vi "PC Fish Control.vi"() -> ()   [LabVIEW 2014]
uses:
  <vilib>/Instr/_visa.llb/VISA Flush IO Buffer Mask.ctl
panel:
  in  "Tab Control":T1(tab)
  in  "Fish Communication Network\nVISA Port":refnum<visa-resource-name>="COM6"
  in  "GPS Network\nVISA Port":refnum<visa-resource-name>="COM8"
  in  "Fish Communication Network\nError In":errorcluster
  in  "GPS Network\nError In":errorcluster
  out "GPS Network \nHandshake Successful?":bool
  out "Comms Network \nHandshake Successful?":bool
  out "Handshake Complete":bool
  out "Handshake Aborted":bool
  in  "MHeading":i32(slide) scale=-45.0..45.0
  in  "MSpeed":i32(slide) scale=-50.0..50.0
  in  "Command Selection":string(combo)="0"
  out "Currently Transmitting\nComms Input":string
  in  "GPS Input":string="C, 400, 300 175"
  out "Currently Transmitting \nGPS Input":string
  out "Running?":bool
  in  "stop":bool caption="ESTOP"
  out "error out":errorcluster
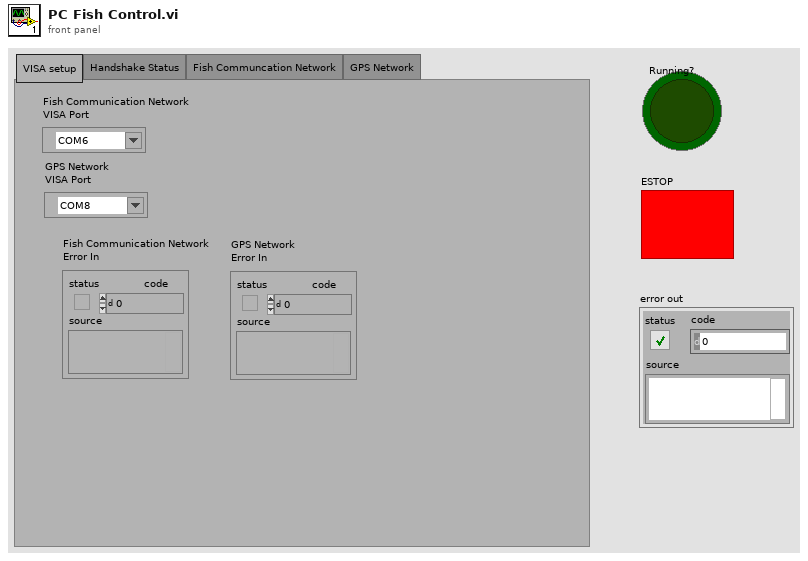
[diagram p1: front panel]
types:
  T1 = enum32{"VISA setup", "Handshake Status", "Fish Communcation Network", "GPS Network"}
  T2 = typedef "VISA Flush IO Buffer Mask.ctl" = u16
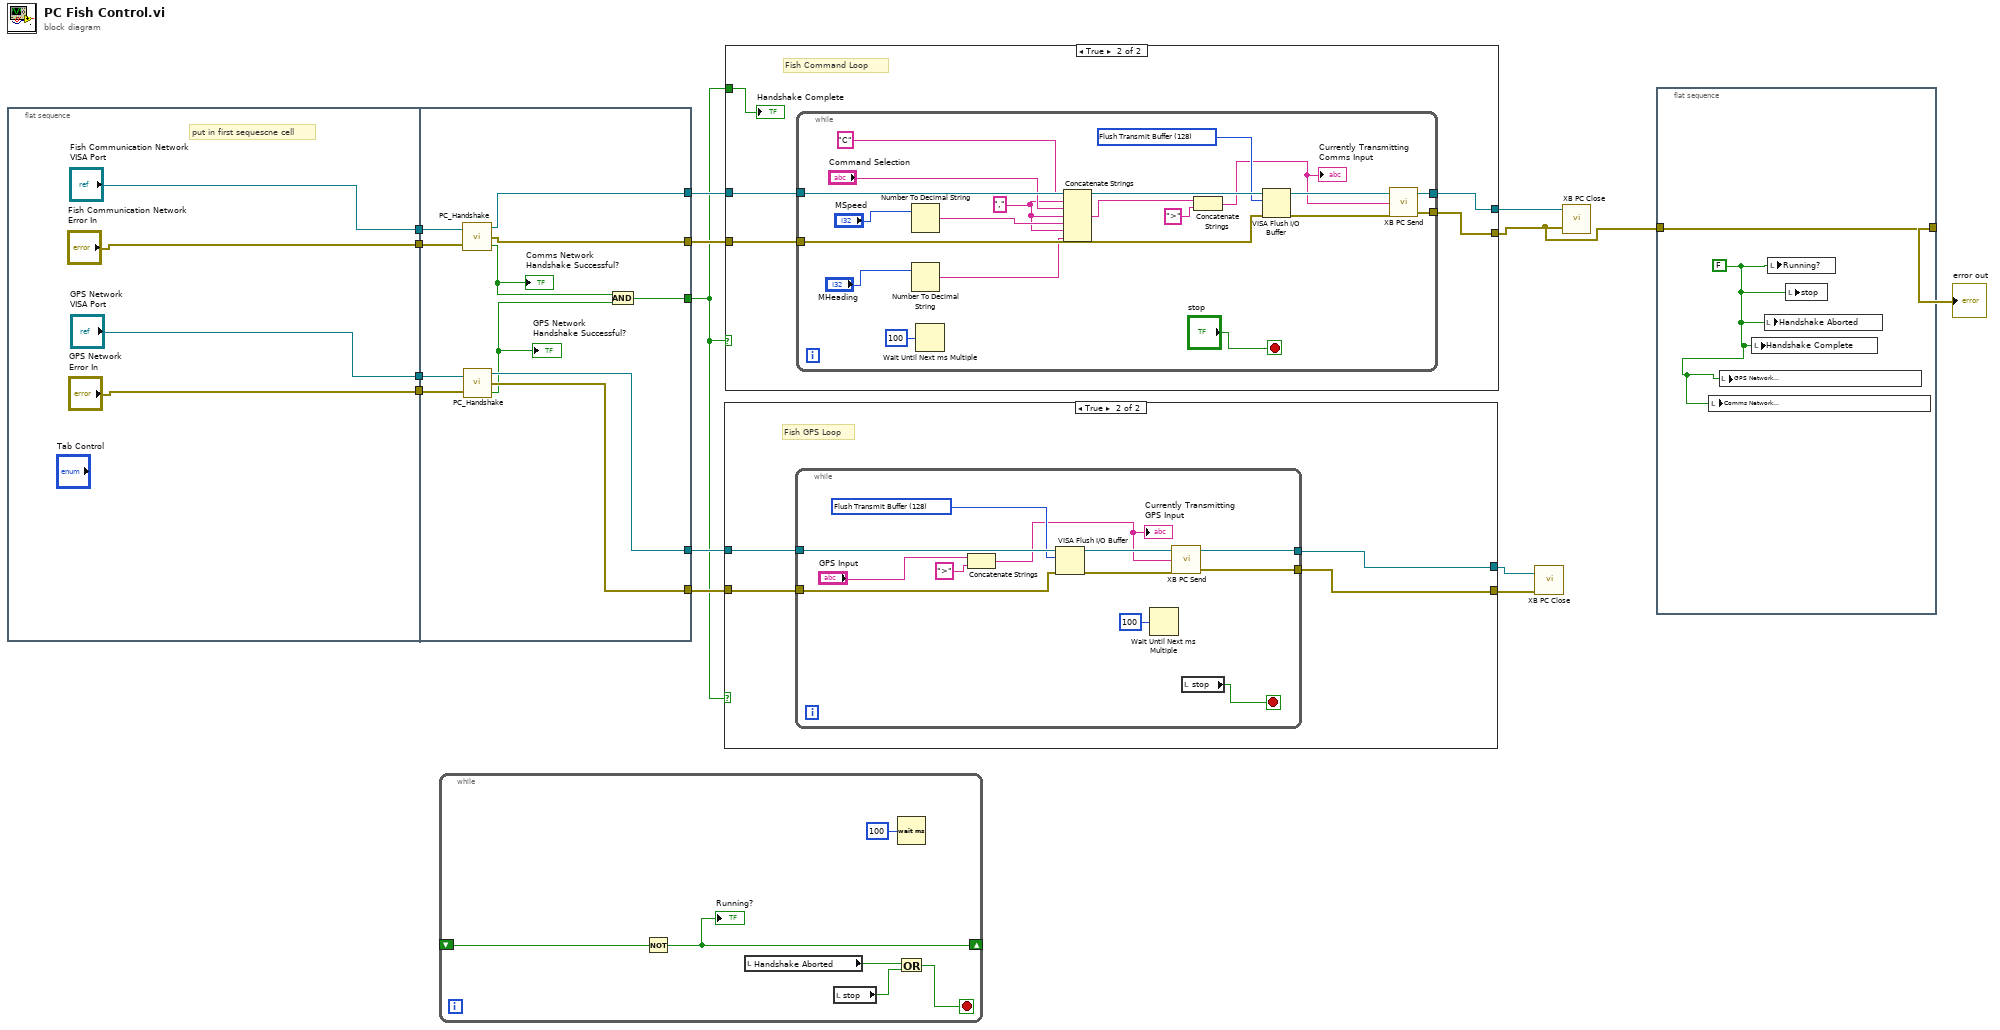
[diagram p0: block diagram]
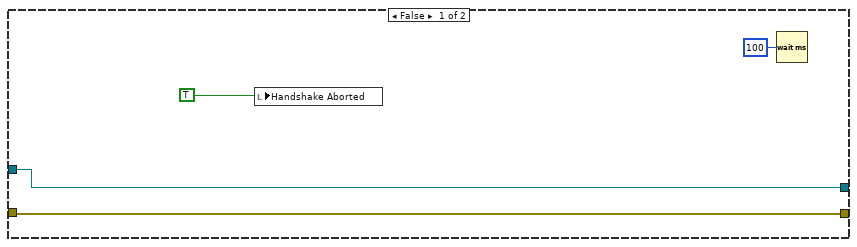
[diagram p2: hidden frame]
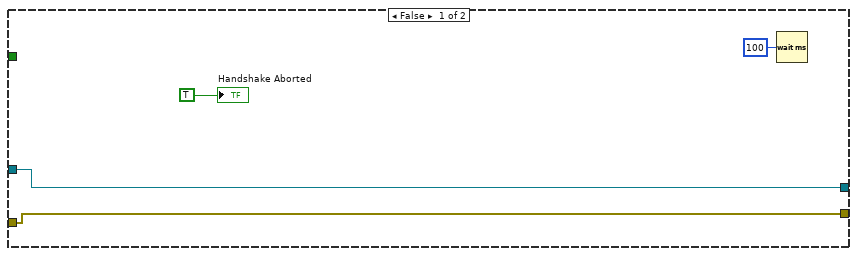
[diagram p3: hidden frame]
diagram:
  n1 = flat-sequence {
    tunnel: ["Fish Communication Network\nVISA Port"] -> w9
    tunnel: ["Fish Communication Network\nError In"] -> w8
    tunnel: ["GPS Network\nVISA Port"] -> w7
    tunnel: ["GPS Network\nError In"] -> w6
    tunnel: w9 -> [w29]
    tunnel: w8 -> [w28]
    tunnel: w7 -> [w27]
    tunnel: w6 -> [w26]
    tunnel: [w25] -> w5
    tunnel: [w24] -> w4
    tunnel: [w23] -> w3
    tunnel: [w22] -> w2
    tunnel: [w21] -> w1
    frame #0 {
      # "put in first sequescne cell"
    }
    frame #1 {
      n2 = call "PC_Handshake.vi"("VISA resource name"=w29, "error in"=w28) -> ("VISA resource name out"=w25:refnum<visa-resource-name>, "error out"=w24:errorcluster, "Handshake Successful?"=w19:bool)
      "Comms Network \nHandshake Successful?" <- w19
      n3 = call "PC_Handshake.vi"("VISA resource name"=w27, "error in"=w26) -> ("VISA resource name out"=w23:refnum<visa-resource-name>, "error out"=w22:errorcluster, "Handshake Successful?"=w20:bool)
      "GPS Network \nHandshake Successful?" <- w20
      n4 = And(x=w19, y=w20) -> (x .and. y?=w21:bool)
    }
  }
  n5 = while {
    shift-right: [w34] -> _
    shift-left: _ -> [w35]
    stop <- w32 stop-if-true
    n6 = Not(x=w35) -> (.not. x?=w34:bool)
    "Running?" <- w34
    n7 = local read "Handshake Aborted"() -> (w30:bool)
    n8 = local read "stop"() -> (w31:bool)
    n9 = Wait (ms)(milliseconds to wait=u32 100) -> ()  [unwired: 1 out]
    n10 = Or(x=w30, y=w31) -> (x .or. y?=w32:bool)
  }
  n11 = case shown="True" w1 {
    tunnel: w3 -> [w38 w43]
    tunnel: w2 -> [w37 w42]
    tunnel: [w38 w41] -> w12
    tunnel: [w37 w40] -> w11
    frame False {
      n12 = local write "Handshake Aborted"(TRUE) -> ()
      n13 = Wait (ms)(milliseconds to wait=u32 100) -> ()  [unwired: 1 out]
    }
    frame True {
      # "Fish GPS Loop"
      n14 = while {
        tunnel: w43 -> [w52]
        tunnel: w42 -> [w50]
        tunnel: [w53] -> w40
        tunnel: [w54] -> w41
        stop <- w45 stop-if-true
        w48 = T2 128 items=["Flush Receive Buffer"=16, "Write Transmit Buffer to Device"=32, "Flush Receive Buffer (No I/O)"=64, "Flush Transmit Buffer"=128] ("Mask")
        n15 = Concatenate Strings("GPS Input", ">" ("string")) -> (w46:string)
        "Currently Transmitting \nGPS Input" <- w46
        n16 = VISA Flush I/O Buffer(VISA resource name=w52, mask (16)=w48, error in (no error)=w50) -> (VISA resource name out=w51:refnum<visa-resource-name>, error out=w49:errorcluster)
        n17 = Wait Until Next ms Multiple(millisecond multiple=u32 100) -> ()  [unwired: 1 out]
        n18 = call "XB PC Send.vi"("error in (no error)"=w49, "String"=w46, "VISA resource name"=w51) -> ("error out"=w53:errorcluster, "VISA resource name out"=w54:refnum<visa-resource-name>)  [unwired: 1 out]
        n19 = local read "stop"() -> (w45:bool)
      }
    }
  }
  n20 = case shown="True" w1 {
    tunnel: w5 -> [w57 w64]
    tunnel: w1 -> [_ w61]
    tunnel: [w57 w63] -> w14
    tunnel: [w56 w62] -> w10
    tunnel: w4 -> [w56 w60]
    frame False {
      n21 = Wait (ms)(milliseconds to wait=u32 100) -> ()  [unwired: 1 out]
      "Handshake Aborted" <- TRUE
    }
    frame True {
      # "Fish Command Loop"
      n22 = while {
        tunnel: w64 -> [w79]
        tunnel: w60 -> [w77]
        tunnel: [w80] -> w62
        tunnel: [w81] -> w63
        stop <- "stop" stop-if-true
        w65 = "," ("string")
        w75 = T2 128 items=["Flush Receive Buffer"=16, "Write Transmit Buffer to Device"=32, "Flush Receive Buffer (No I/O)"=64, "Flush Transmit Buffer"=128] ("Mask")
        n23 = Number To Decimal String(number="MSpeed") -> (decimal integer string=w68:string)  [unwired: 1 in]
        n24 = Number To Decimal String(number="MHeading") -> (decimal integer string=w67:string)  [unwired: 1 in]
        n25 = Wait Until Next ms Multiple(millisecond multiple=u32 100) -> ()  [unwired: 1 out]
        n26 = Concatenate Strings("C" ("string"), w65, "Command Selection", w65, w68, w65, w67) -> (w69:string)
        n27 = Concatenate Strings(w69, ">" ("string")) -> (w74:string)
        "Currently Transmitting\nComms Input" <- w74
        n28 = VISA Flush I/O Buffer(VISA resource name=w79, mask (16)=w75, error in (no error)=w77) -> (VISA resource name out=w78:refnum<visa-resource-name>, error out=w76:errorcluster)
        n29 = call "XB PC Send.vi"("error in (no error)"=w76, "String"=w74, "VISA resource name"=w78) -> ("error out"=w80:errorcluster, "VISA resource name out"=w81:refnum<visa-resource-name>)  [unwired: 1 out]
      }
      "Handshake Complete" <- w61
    }
  }
  n30 = call "XB PC Close.vi"("error in (no error)"=w11, "VISA resource name"=w12) -> ()
  n31 = call "XB PC Close.vi"("error in (no error)"=w10, "VISA resource name"=w14) -> ()
  n32 = flat-sequence {
    tunnel: w10 -> [w85]
    tunnel: [w85] -> w13
    frame #0 {
      w84 = FALSE
      n33 = local write "Comms Network \nHandshake Successful?"(w84) -> ()
      n34 = local write "GPS Network \nHandshake Successful?"(w84) -> ()
      n35 = local write "Handshake Complete"(w84) -> ()
      n36 = local write "Handshake Aborted"(w84) -> ()
      n37 = local write "Running?"(w84) -> ()
      n38 = local write "stop"(w84) -> ()
    }
  }
  "error out" <- w13
